vi "unqualify channel.vi"(10 "qualified channel":refnum<class "TBM channel.lvclass">, 11 "module configuration in":refnum<class "TBM module configuration.lvclass">) -> (2 "unqualified channel":refnum<class "TBM channel.lvclass">, 3 "module configuration out":refnum<class "TBM module configuration.lvclass">)   [LabVIEW 2013, in "TBM module configuration.lvclass"]
doc: "Converts a qualified channel into an unqualified channel, based on the rules of the module."
uses:
  TBM module configuration.lvclass
  channel/TBM channel.lvclass
  <vilib>/NI/Tag Bus/tag/tag descriptor.lvclass/tag descriptor.ctl
  <vilib>/NI/Configuration Framework/serializable configuration/NISE_CEF_serializable configuration.lvclass/NISE_CEF_serializable configuration.ctl
  <vilib>/NI/Configuration Framework/serializable configuration/NISE_CEF_serializable configuration.lvclass
  <vilib>/NI/Tag Bus/tag/tag descriptor.lvclass
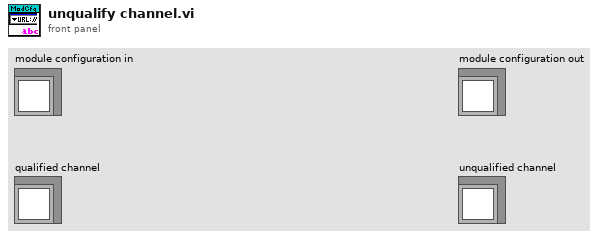
[diagram p1: front panel]
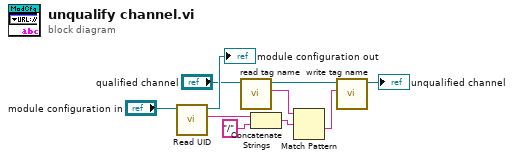
[diagram p0: block diagram]
diagram:
  n1 = call <vilib>:"Read UID.vi"("configuration in"="module configuration in") -> ("instance id"=w6:string, "configuration out"=→"module configuration out":refnum<class "TBM module configuration.lvclass">)  [unwired: 8 in, 1 out]
  n2 = call <vilib>:"read tag name.vi"("system tag in"="qualified channel") -> ("name"=w3:string, "system tag out"=w9:refnum<class "TBM channel.lvclass">)  [unwired: 8 in, 1 out]
  n3 = Concatenate Strings(w6, "/" ("string")) -> (w1:string)
  n4 = Match Pattern(string=w3, regular expression=w1) -> (after substring=w2:string)  [unwired: 1 in, 3 out]
  n5 = call <vilib>:"write tag name.vi"("name"=w2, "system tag in"=w9) -> ("system tag out"=→"unqualified channel":refnum<class "TBM channel.lvclass">)  [unwired: 8 in, 1 out]
